vi "EMV Calculate T6 minus Setpont Upper Lower Limits.vi"(8 "error in (no error)":errorcluster, 10 "Sigma":dbl=4.0 format="%#_13g", 11 "T6-Setpoint":dbl) -> (0 "error out":errorcluster, 2 "Lower Limit":dbl, 3 "Upper Limit":dbl)   [LabVIEW 2020]
uses:
  <vilib>/ptbypt/NI_PtbyPt.lvlib
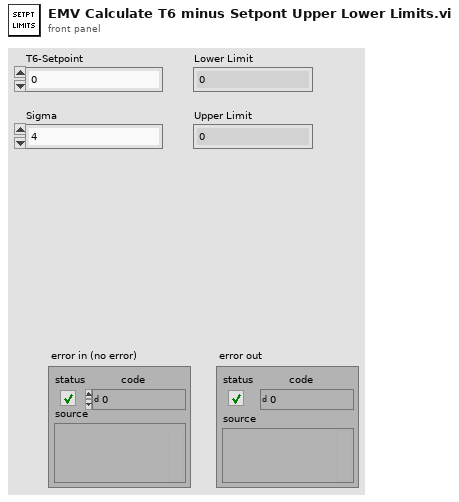
[diagram p1: front panel]
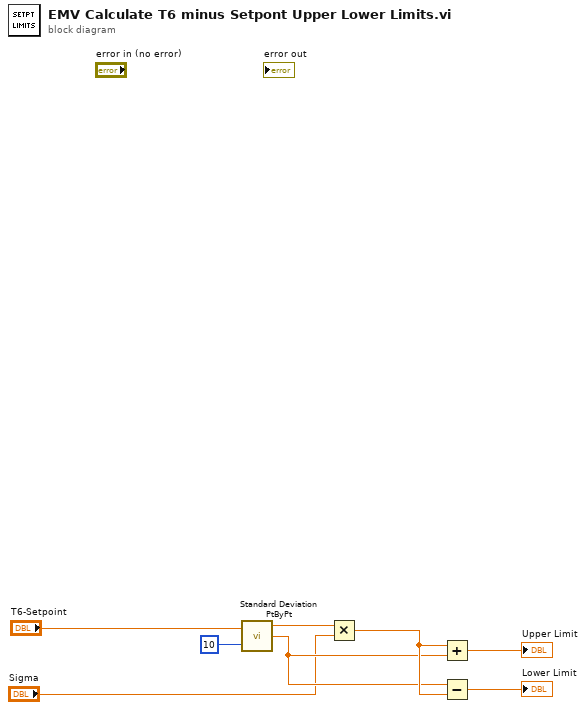
[diagram p0: block diagram]
diagram:
  n1 = call <vilib>:"Standard Deviation PtByPt.vi"("x"="T6-Setpoint", "sample length"=10) -> ("standard deviation"=w3:dbl, "mean"=w4:dbl)  [unwired: 1 in, 1 out]
  n2 = Multiply(x=w3, y="Sigma") -> (x*y=w5:dbl)
  n3 = Add(x=w5, y=w4) -> (x+y=→"Upper Limit":dbl)
  n4 = Subtract(x=w4, y=w5) -> (x-y=→"Lower Limit":dbl)
